vi "Main PC.vi"() -> ()   [LabVIEW 2021]
uses:
  IP addresses.lvlib
panel:
  out "IPs availables":i32
  out "IP/Domains":string[](array[string])
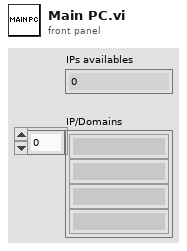
[diagram p1: front panel]
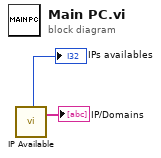
[diagram p0: block diagram]
diagram:
  n1 = call "IP Available.vi"() -> ("IPs availables"=→"IPs availables":i32, "IP/Domain"=→"IP/Domains":string[])  [unwired: 4 in]
